vi "Initialize.vi"(8 "error in (no error)":errorcluster, 11 "Stage in":refnum<class "Stage.lvclass">) -> (0 "error out":errorcluster, 3 "Stage out":refnum<class "Stage.lvclass">)   [LabVIEW 2020, in "Stage.lvlib" / "Stage.lvclass"]
uses:
  Stage.lvclass
  Device/Device/Device.lvclass
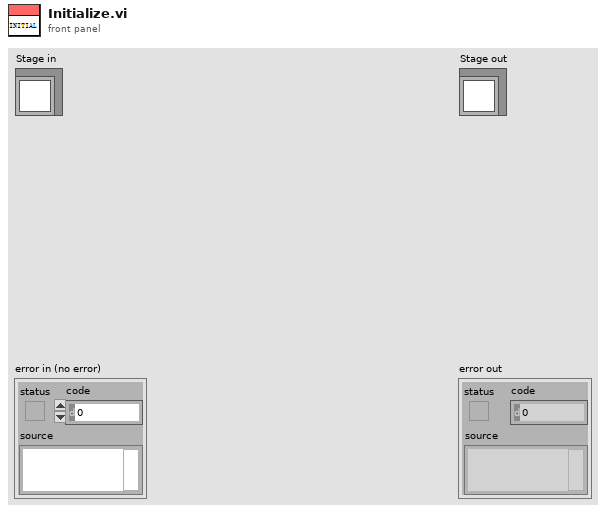
[diagram p1: front panel]
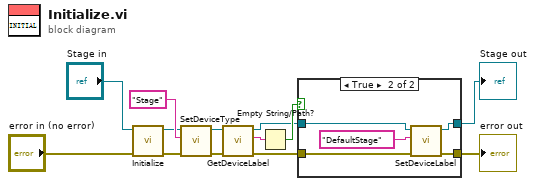
[diagram p0: block diagram]
diagram:
  n1 = call-parent "Initialize.vi"("error in (no error)"="error in (no error)", "Device in"="Stage in") -> ("error out"=w4:errorcluster, "Device out"=w3:refnum<class "Stage.lvclass">)  [unwired: 8 in]
  n2 = call-dynamic "SetDeviceType.vi"("error in (no error)"=w4, "Type"="Stage", "Device in"=w3) -> ("error out"=w11:errorcluster, "Device out"=w9:refnum<class "Stage.lvclass">)  [unwired: 7 in]
  n3 = call-dynamic "GetDeviceLabel.vi"("error in (no error)"=w11, "Device in"=w9) -> ("error out"=w5:errorcluster, "Label"=w8:string, "Device out"=w6:refnum<class "Stage.lvclass">)  [unwired: 7 in]
  n4 = Empty String/Path?(string/path=w8) -> (empty?=w7:bool)
  n5 = case shown="True" w7 {
    tunnel: w6 -> [w15 w18]
    tunnel: w5 -> [w14 w20]
    tunnel: [w15 w17] -> w2
    tunnel: [w14 w19] -> w1
    frame False {
    }
    frame True {
      n6 = call-dynamic "SetDeviceLabel.vi"("error in (no error)"=w20, "Label"="DefaultStage", "Device in"=w18) -> ("error out"=w19:errorcluster, "Device out"=w17:refnum<class "Stage.lvclass">)  [unwired: 7 in]
    }
  }
  "error out" <- w1
  "Stage out" <- w2
